vi "FollowADottedLine.vi"   [LabVIEW 2016, in "LEGO-PMR.lvrbt"]
uses:
  LEGO-PMR.lvrbt
  <vilib>/NXT/Block Support/NXT_InputPort.ctl
  <vilib>/NXT/Block Support/NXT_OutputPort.ctl
  <vilib>/NXT/Dual Mode Library/Sensors/EV3_Color_Reflect.vi
  <vilib>/NXT/Dual Mode Library/Waits/Wait_Num(msec).vi
  <vilib>/NXT/NXTIO Xnodes/NXTIONodeSubVIs/NXTMoveMotors.vi
  <vilib>/NXT/NXTIO Xnodes/AddressXNode/NXTIOAddress.xnode
  <vilib>/NXT/Subs/LVHSConnector.ctl
  <vilib>/NXT/NXTIO Xnodes/NXTIOXNode/NXTIO.xnode
  <vilib>/NXT/LegoClasses/BrickReference/BrickReference.lvclass
types:
  T1 = typedef "NXT_InputPort.ctl" = u32
  T2 = typedef "NXT_OutputPort.ctl" = u8
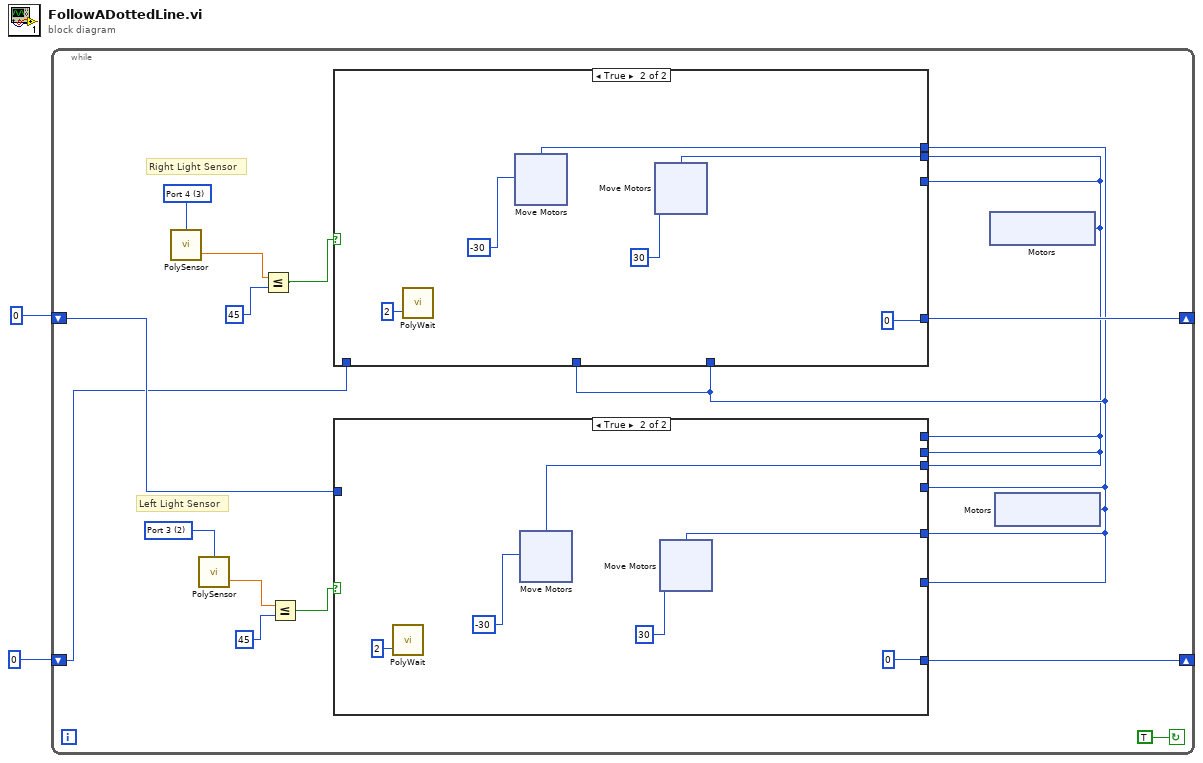
[diagram p0: block diagram]
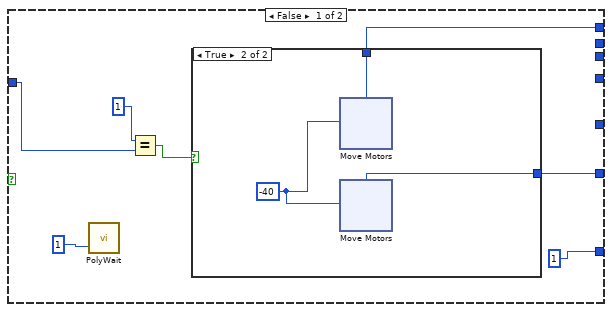
[diagram p2: hidden frame]
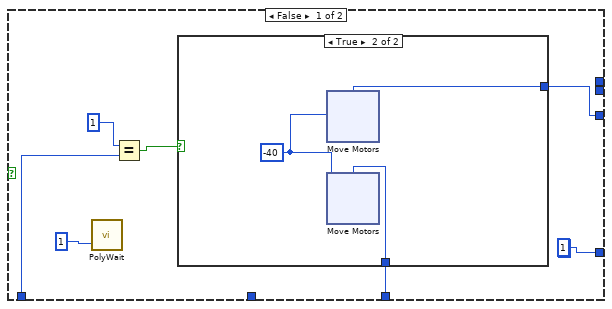
[diagram p4: hidden frame]
diagram:
  n1 = while {
    shift-right: [w8] -> _
    shift-left: 0 -> [w6]
    shift-right: [w7] -> _
    shift-left: 0 -> [w5]
    stop <- TRUE continue-if-true
    w16 = T1 3 items=["Port 1", "Port 2", "Port 3", "Port 4"] ("Port (Port 1)")
    w17 = T1 2 items=["Port 1", "Port 2", "Port 3", "Port 4"] ("Port (Port 1)")
    # "Left Light Sensor"
    # "Right Light Sensor"
    n2 = call-poly <vilib>:"PolySensor.vi"("Port (Port 1)"=w16) -> ("Scaled Value"=w13:sgl)  [unwired: 2 in, 1 out]
    n3 = call-poly <vilib>:"PolySensor.vi"("Port (Port 1)"=w17) -> ("Scaled Value"=w11:sgl)  [unwired: 2 in, 1 out]
    n4 = Less Or Equal?(x=w13, y=45) -> (x <= y?=w14:bool)
    n5 = Less Or Equal?(x=w11, y=45) -> (x <= y?=w9:bool)
    n6 = xnode "Motors"() -> ("Motor"=w3:T2)
    n7 = xnode "Motors"() -> ("Motor"=w4:T2)
    n8 = case shown="True" w14 {
      tunnel: w3 -> [w66 _]
      tunnel: w4 -> [_ _]
      tunnel: [1 0] -> w8
      tunnel: w5 -> [w69 _]
      tunnel: w4 -> [w65 _]
      tunnel: w3 -> [_ w90]
      tunnel: w4 -> [_ w89]
      frame False {
        (unwired) 1
        n9 = call-poly <vilib>:"PolyWait.vi"("Time (100 msec)"=u32 1) -> ()  [unwired: 3 in, 1 out]
        n10 = Equal?(x=1, y=w69) -> (x = y?=w67:bool)
        n11 = case shown="True" w67 {
          tunnel: w66 -> [_ w72]
          tunnel: w65 -> [_ w71]
          frame False {
          }
          frame True {
            w73 = -40
            n12 = xnode "Move Motors"("Power/Speed 1"=w73, "Motors"=w72) -> ()  [unwired: 1 in, 1 out]
            n13 = xnode "Move Motors"("Power/Speed 1"=w73, "Motors"=w71) -> ()  [unwired: 1 in, 1 out]
          }
        }
      }
      frame True {
        n14 = call-poly <vilib>:"PolyWait.vi"("Time (100 msec)"=u32 2) -> ()  [unwired: 3 in, 1 out]
        n15 = xnode "Move Motors"("Power/Speed 1"=-30, "Motors"=w89) -> ()  [unwired: 1 in, 1 out]
        n16 = xnode "Move Motors"("Power/Speed 1"=30, "Motors"=w90) -> ()  [unwired: 1 in, 1 out]
      }
    }
    n17 = case shown="True" w9 {
      tunnel: w3 -> [_ _]
      tunnel: w4 -> [_ _]
      tunnel: [1 0] -> w7
      tunnel: w6 -> [w25 _]
      tunnel: w3 -> [w22 _]
      tunnel: w4 -> [w21 _]
      tunnel: w4 -> [_ w46]
      tunnel: w3 -> [_ w45]
      frame False {
        n18 = call-poly <vilib>:"PolyWait.vi"("Time (100 msec)"=u32 1) -> ()  [unwired: 3 in, 1 out]
        n19 = Equal?(x=1, y=w25) -> (x = y?=w23:bool)
        n20 = case shown="True" w23 {
          tunnel: w22 -> [_ w28]
          tunnel: w21 -> [_ w27]
          frame False {
          }
          frame True {
            w29 = -40
            n21 = xnode "Move Motors"("Power/Speed 1"=w29, "Motors"=w28) -> ()  [unwired: 1 in, 1 out]
            n22 = xnode "Move Motors"("Power/Speed 1"=w29, "Motors"=w27) -> ()  [unwired: 1 in, 1 out]
          }
        }
      }
      frame True {
        n23 = call-poly <vilib>:"PolyWait.vi"("Time (100 msec)"=u32 2) -> ()  [unwired: 3 in, 1 out]
        n24 = xnode "Move Motors"("Power/Speed 1"=-30, "Motors"=w45) -> ()  [unwired: 1 in, 1 out]
        n25 = xnode "Move Motors"("Power/Speed 1"=30, "Motors"=w46) -> ()  [unwired: 1 in, 1 out]
      }
    }
  }
